vi "InterfazControlador.vi"() -> ()   [LabVIEW 2013]
uses:
  <vilib>/Instr/_visa.llb/VISA Configure Serial Port (Instr).vi
panel:
  in  "Paro":bool
  in  "Iniciar Transmisión":bool
  in  "Start":bool
  in  "Referencia de altura [cm]":u8(knob) scale=0.0..200.0
  out "Datos enviados":string
  in  "stop":bool
  out "Datos recibidos":string
  in  "Puerto Serial":refnum<visa-resource-name>
  # "Programa para calibrar y probar los motores brushless"
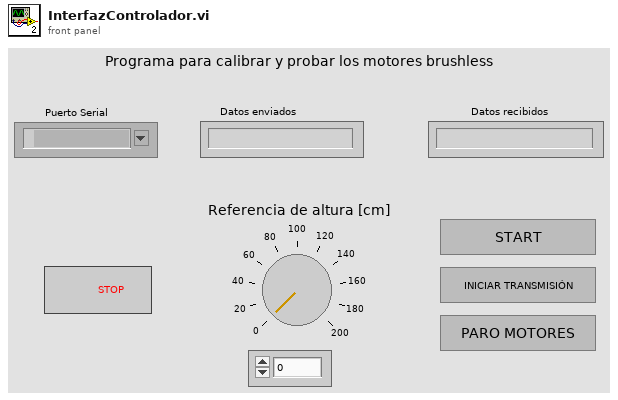
[diagram p1: front panel]
types:
  T1 = enum16{"INICIO", "INIT", "LOOP", "DETENER", "FIN"}
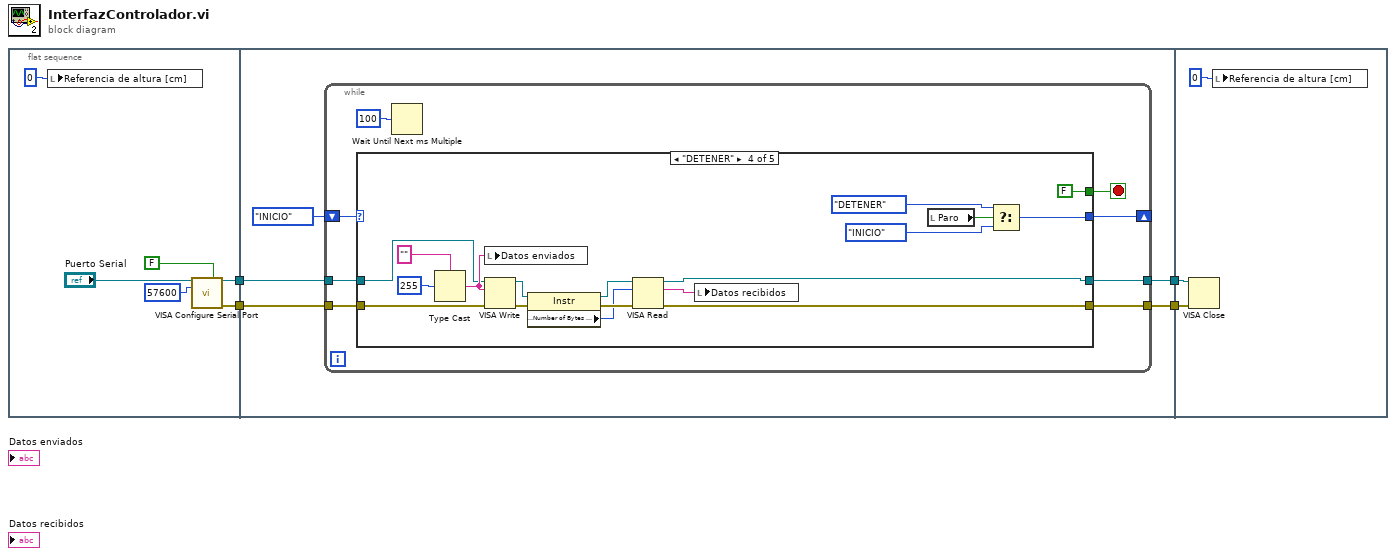
[diagram p0: block diagram]
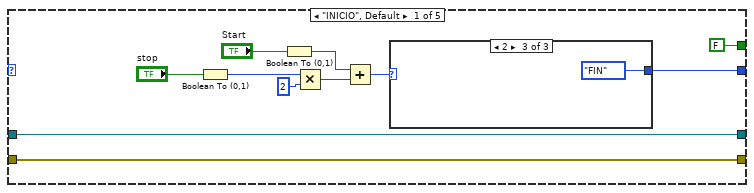
[diagram p2: hidden frame]
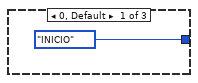
[diagram p3: hidden frame]
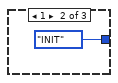
[diagram p4: hidden frame]
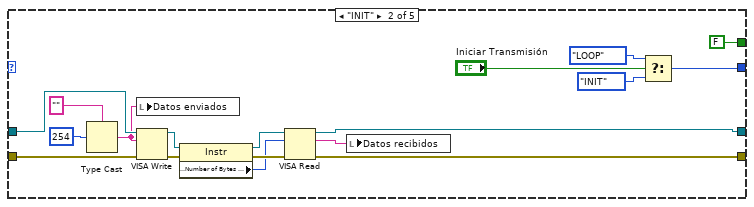
[diagram p5: hidden frame]
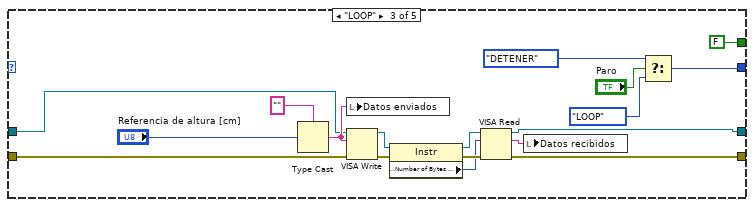
[diagram p6: hidden frame]
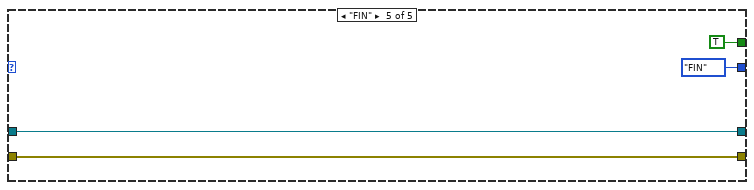
[diagram p7: hidden frame]
diagram:
  n1 = flat-sequence {
    tunnel: [w8] -> w4
    tunnel: [w7] -> w3
    tunnel: w4 -> [w14]
    tunnel: w3 -> [w12]
    tunnel: [w13] -> w2
    tunnel: [w11] -> w1
    tunnel: w2 -> [w97]
    tunnel: w1 -> [w96]
    frame #0 {
      n2 = local write "Referencia de altura [cm]"(u8 0 ("Dial")) -> ()
      n3 = call-poly "VISA Configure Serial Port"("VISA resource name"="Puerto Serial", "Enable Termination\nChar (T)"=FALSE ("Enable Termination\nChar (T)"), "baud rate (9600)"=u32 57600) -> ("VISA resource name out"=w8:refnum<visa-resource-name>, "error out"=w7:errorcluster)  [unwired: 11 in]
    }
    frame #1 {
      n4 = while {
        shift-right: [w22] -> _
        shift-left: T1."INICIO" -> [w23]
        tunnel: w14 -> [w19]
        tunnel: [w18] -> w13
        tunnel: w12 -> [w17]
        tunnel: [w16] -> w11
        stop <- w20 stop-if-true
        n5 = case shown="\"DETENER\"" w23 {
          tunnel: [w26 w53 w71 w89 T1."FIN"] -> w22
          tunnel: [FALSE FALSE FALSE FALSE TRUE] -> w20
          tunnel: w19 -> [w25 w45 w59 w77 w93]
          tunnel: [w25 w39 w57 w75 w93] -> w18
          tunnel: w17 -> [w24 w44 w58 w76 w92]
          tunnel: [w24 w38 w56 w74 w92] -> w16
          frame "INICIO", Default {
            n6 = Boolean To (0,1)(Boolean="stop") -> (0, 1=w30:i16)
            n7 = Boolean To (0,1)(Boolean="Start") -> (0, 1=w31:i16)
            n8 = Multiply(x=w30, y=i16 2) -> (x*y=w28:i16)
            n9 = Add(x=w31, y=w28) -> (x+y=w27:i16)
            n10 = case shown="2" w27 {
              tunnel: [T1."INICIO" T1."INIT" T1."FIN"] -> w26
              frame 0, Default {
              }
              frame 1 {
              }
              frame 2 {
              }
            }
          }
          frame "INIT" {
            n11 = Type Cast(type="", x=u32 254 ("millisecond multiple")) -> (*(type *) &x=w41:string)
            n12 = local write "Datos enviados"(w41) -> ()
            n13 = VISA Write(VISA resource name=w45, write buffer=w41, error in (no error)=w44) -> (VISA resource name out=w47:refnum<visa-resource-name>, error out=w46:errorcluster)  [unwired: 1 out]
            n14 = property class="Instr"(reference=w47, error in=w46) -> (reference out=w48:refnum<visa-resource-name>, error out=w50:errorcluster, "Serial Settings:Number of Bytes at Serial Port"=w49:u32)
            n15 = VISA Read(VISA resource name=w48, byte count=w49, error in (no error)=w50) -> (VISA resource name out=w39:refnum<visa-resource-name>, read buffer=w40:string, error out=w38:errorcluster)  [unwired: 1 out]
            n16 = local write "Datos recibidos"(w40) -> ()
            n17 = Select(t=T1."LOOP", s="Iniciar Transmisión", f=T1."INIT") -> (s? t:f=w53:T1)
          }
          frame "LOOP" {
            n18 = Type Cast(type="", x="Referencia de altura [cm]") -> (*(type *) &x=w63:string)
            n19 = local write "Datos enviados"(w63) -> ()
            n20 = VISA Write(VISA resource name=w59, write buffer=w63, error in (no error)=w58) -> (VISA resource name out=w65:refnum<visa-resource-name>, error out=w64:errorcluster)  [unwired: 1 out]
            n21 = property class="Instr"(reference=w65, error in=w64) -> (reference out=w66:refnum<visa-resource-name>, error out=w68:errorcluster, "Serial Settings:Number of Bytes at Serial Port"=w67:u32)
            n22 = VISA Read(VISA resource name=w66, byte count=w67, error in (no error)=w68) -> (VISA resource name out=w57:refnum<visa-resource-name>, read buffer=w62:string, error out=w56:errorcluster)  [unwired: 1 out]
            n23 = local write "Datos recibidos"(w62) -> ()
            n24 = Select(t=T1."DETENER", s="Paro", f=T1."LOOP") -> (s? t:f=w71:T1)
          }
          frame "DETENER" {
            n25 = Type Cast(type="", x=u32 255 ("millisecond multiple")) -> (*(type *) &x=w79:string)
            n26 = local write "Datos enviados"(w79) -> ()
            n27 = VISA Write(VISA resource name=w77, write buffer=w79, error in (no error)=w76) -> (VISA resource name out=w83:refnum<visa-resource-name>, error out=w82:errorcluster)  [unwired: 1 out]
            n28 = property class="Instr"(reference=w83, error in=w82) -> (reference out=w84:refnum<visa-resource-name>, error out=w86:errorcluster, "Serial Settings:Number of Bytes at Serial Port"=w85:u32)
            n29 = VISA Read(VISA resource name=w84, byte count=w85, error in (no error)=w86) -> (VISA resource name out=w75:refnum<visa-resource-name>, read buffer=w78:string, error out=w74:errorcluster)  [unwired: 1 out]
            n30 = local write "Datos recibidos"(w78) -> ()
            n31 = local read "Paro"() -> (w88:bool)
            n32 = Select(t=T1."DETENER", s=w88, f=T1."INICIO") -> (s? t:f=w89:T1)
          }
          frame "FIN" {
          }
        }
        n33 = Wait Until Next ms Multiple(millisecond multiple=u32 100) -> ()  [unwired: 1 out]
      }
    }
    frame #2 {
      n34 = VISA Close(VISA resource name=w97, error in (no error)=w96) -> ()  [unwired: 1 out]
      n35 = local write "Referencia de altura [cm]"(u8 0 ("Dial")) -> ()
    }
  }
